vi "wait autonomous (WHS-ROB-6PZCBS1's conflicted copy 2013-02-20).vi"() -> ()   [LabVIEW 2010, in "Rampage.lvrbt"]
uses:
  Rampage.lvrbt
  <vilib>/NXT/Subs/MotorOutput.ctl
  <vilib>/NXT/NXTIO Xnodes/AddressXNode/NXTIOAddress.xnode
  <vilib>/NXT/Subs/MotorXNode.DC Motor Type.ctl
  <vilib>/NXT/Subs/MotorXNode.2DCMotor.ctl
  <vilib>/NXT/HiTechnic/HiTechnic Controls/HiTechnic Port.ctl
  <vilib>/NXT/Block Support/NXT_InputPort.ctl
  <vilib>/NXT/NXTIO Xnodes/NXTIOXNode/NXTIO.xnode
  <vilib>/NXT/Subs/LVHSConnector.ctl
  <vilib>/NXT/Dual Mode Library/Waits/Wait_Num(msec).vi
  <vilib>/NXT/Dual Mode Library/prims/inRangeAndCoerce/inRangeAndCoerce_int.vi
  <vilib>/NXT/Dual Mode Library/Motors/MotorOn.vi
  <vilib>/NXT/Dual Mode Library/Waits/Wait_Num.vi
  <vilib>/NXT/NXTIO Xnodes/NXTIONodeSubVIs/TETRIX IO Move DC Motors.vi
  <vilib>/NXT/NXTIO Xnodes/NXTIONodeSubVIs/TETRIX IO Stop DC Motors.vi
  <vilib>/NXT/Dual Mode Library/Sensors/Sonar_cm.vi
panel:
  out "Enabled":bool
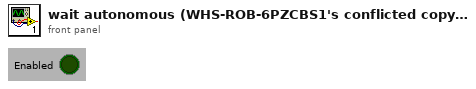
[diagram p1: front panel]
types:
  T1 = typedef "LVHSConnector.ctl" = cluster{"Hardware":string, "Flattened String":string}
  T2 = typedef "MotorOutput.ctl" = u8
  T3 = typedef "MotorXNode.DC Motor Type.ctl" = enum16{"DC Motor"}
  T4 = cluster{"DC Motor":T3, "Address":i16, "Address":i16}
  T5 = typedef "HiTechnic Port.ctl" = cluster{"Port":T6, "MUX Port":u8}
  T6 = typedef "NXT_InputPort.ctl" = u8
  T7 = cluster{"Direction (0-9)":i16, "Signal Strength (Array)":u8[]}
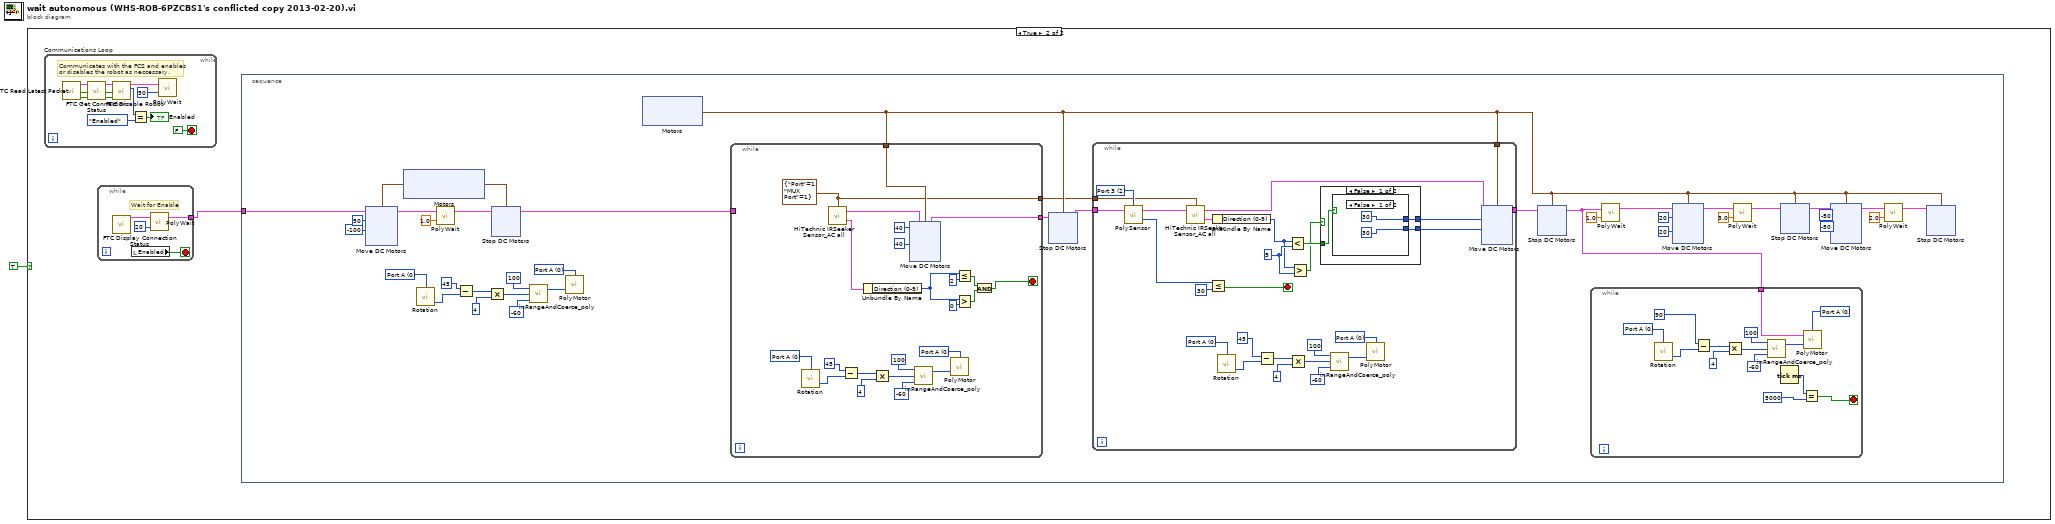
[diagram p0: block diagram]
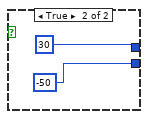
[diagram p3: hidden frame]
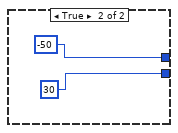
[diagram p4: hidden frame]
diagram:
  n1 = case shown="True" TRUE {
    frame False {
    }
    frame True {
      n2 = while "Communications Loop" {
        stop <- FALSE stop-if-true
        # "Communicates with the FCS and enables \nor disables the robot as neccessary."
        n3 = call <vilib>:"FTC Read Latest Packet.vi"() -> ("Packet Received?"=w213:bool, "Stopped?"=w212:bool, "NXT"=w215:T1)  [unwired: 6 in, 3 out]
        n4 = call <vilib>:"FTC Get Connection Status.vi"("Packet Received?"=w213, "Stopped?"=w212, "NXT"=w215) -> ("Online?"=w204:bool, "Stopped?"=w205:bool, "NXT"=w214:T1)  [unwired: 5 in]
        n5 = call <vilib>:"FTC Disable Robot.vi"("Online?"=w204, "Stopped?"=w205, "NXT"=w214) -> ("Enabled?"=w208:enum16{"Disabled", "Enabled"}, "NXT"=w210:T1)  [unwired: 3 in]
        n6 = Equal?(x=w208, y=enum16{"Disabled", "Enabled"}."Enabled") -> (x = y?=→"Enabled":bool)
        n7 = call-poly <vilib>:"PolyWait.vi"("Time (100 msec)"=u32 50 ("Time (msec)"), "NXT"=w210) -> ()  [unwired: 2 in, 1 out]
      }
      n8 = while {
        tunnel: [w201] -> w2
        stop <- w202 stop-if-true
        # "Wait for Enable"
        n9 = call <vilib>:"FTC Display Connection Status.vi"() -> ("NXT"=w200:T1)  [unwired: 11 in]
        n10 = local read "Enabled"() -> (w202:bool)
        n11 = call-poly <vilib>:"PolyWait.vi"("Time (100 msec)"=u32 20 ("Time (msec)"), "NXT"=w200) -> ("NXT"=w201:T1)  [unwired: 2 in]
      }
      n12 = stacked-sequence {
        tunnel: w2 -> [w4]
        frame #0 {
          w31 = T2 0 items=["Port A"=0, "Port B"=1, "Port C"=2, "Ports A & B"=4, "Ports A & C"=5, "Ports B & C"=6, "All Ports"=3] ("Output Port (All Ports)")
          w29 = u8 0 items=["Port A", "Port B", "Port C"] ("Port (Port A)")
          n13 = xnode "Motors"() -> ("DC Motor"=w39:T4)
          n14 = xnode "Move DC Motors"("Power/Speed 1"=i8 50, "Motors"=w39, "NXT"=w4, "Power/Speed 2"=i8 -100) -> ("NXT"=w37:T1)
          n15 = call <vilib>:"Rotation.vi"("Port (Port A)"=w29) -> ("Angle of Rotation"=w32:i32)  [unwired: 2 in, 1 out]
          n16 = call-poly <vilib>:"PolyWait.vi"("Time (1 sec)"=sgl 1.0, "NXT"=w37) -> ("NXT"=w34:T1)  [unwired: 2 in]
          n17 = Subtract(x=45 ("Claw\nPosition"), y=w32) -> (x-y=w30:i32)
          n18 = Multiply(x=w30, y=4) -> (x*y=w28:i32)
          n19 = xnode "Stop DC Motors"("Motors"=w39, "NXT"=w34) -> ("NXT"=w20:T1)
          n20 = call-poly <vilib>:"inRangeAndCoerce_poly.vi"("lower limit"=-60, "x"=w28, "upper limit"=100) -> ("coerced(x)"=w25:i32)  [unwired: 1 out]
          n21 = call-poly <vilib>:"PolyMotor.vi"("Power (75)"=w25, "Output Port (All Ports)"=w31) -> ()  [unwired: 2 in, 1 out]
          n22 = xnode "Motors"() -> ("DC Motor"=w22:T4)
          n23 = while {
            tunnel: [w188] -> w8
            tunnel: w22 -> [w185]
            tunnel: [w172] -> w3
            tunnel: w20 -> [_]
            stop <- w167 stop-if-true
            w177 = T2 0 items=["Port A"=0, "Port B"=1, "Port C"=2, "Ports A & B"=4, "Ports A & C"=5, "Ports B & C"=6, "All Ports"=3] ("Output Port (All Ports)")
            w179 = u8 0 items=["Port A", "Port B", "Port C"] ("Port (Port A)")
            w172 = T5 {"Port"=1, "MUX Port"=1} ("Port/MUX")
            n24 = call <vilib>:"Rotation.vi"("Port (Port A)"=w179) -> ("Angle of Rotation"=w176:i32)  [unwired: 2 in, 1 out]
            n25 = call <vilib>:"HiTechnic IRSeeker Sensor_AC all.vi"("Port/MUX"=w172) -> ("All Info"=w173:T7, "NXT"=w189:T1)  [unwired: 2 in]
            n26 = Subtract(x=45 ("Claw\nPosition"), y=w176) -> (x-y=w178:i32)
            n27 = Unbundle By Name(w173) -> ("Direction (0-9)"=w170:i16)
            n28 = Multiply(x=w178, y=4) -> (x*y=w180:i32)
            n29 = xnode "Move DC Motors"("Power/Speed 2"=i8 40, "Power/Speed 1"=i8 40, "Motors"=w185, "NXT"=w189) -> ("NXT"=w188:T1)
            n30 = call-poly <vilib>:"inRangeAndCoerce_poly.vi"("lower limit"=-60, "x"=w180, "upper limit"=100) -> ("coerced(x)"=w183:i32)  [unwired: 1 out]
            n31 = call-poly <vilib>:"PolyMotor.vi"("Power (75)"=w183, "Output Port (All Ports)"=w177) -> ()  [unwired: 2 in, 1 out]
            n32 = Less Or Equal?(x=w170, y=i16 2) -> (x <= y?=w169:bool)
            n33 = Greater?(x=w170, y=i16 0) -> (0:w168:bool)
            n34 = And(x=w169, y=w168) -> (x .and. y?=w167:bool)
          }
          n35 = xnode "Stop DC Motors"("Motors"=w22, "NXT"=w8) -> ("NXT"=w23:T1)
          n36 = while {
            tunnel: [w138] -> w7
            tunnel: w22 -> [w137]
            tunnel: w23 -> [w115]
            tunnel: w3 -> [w113]
            stop <- w114 stop-if-true
            w118 = T2 0 items=["Port A"=0, "Port B"=1, "Port C"=2, "Ports A & B"=4, "Ports A & C"=5, "Ports B & C"=6, "All Ports"=3] ("Output Port (All Ports)")
            w120 = u8 0 items=["Port A", "Port B", "Port C"] ("Port (Port A)")
            w129 = i16 5 ("y")
            w135 = T6 2 items=["Port 1", "Port 2", "Port 3", "Port 4"] ("Port (Port 4)")
            n37 = call-poly <vilib>:"PolySensor.vi"("NXT"=w115, "Port (Port 4)"=w135) -> ("Distance (cm)"=w136:i16, "NXT"=w134:T1)  [unwired: 1 in]
            n38 = call <vilib>:"HiTechnic IRSeeker Sensor_AC all.vi"("NXT"=w134, "Port/MUX"=w113) -> ("All Info"=w133:T7, "NXT"=w132:T1)  [unwired: 1 in]
            n39 = Less Or Equal?(x=w136, y=i16 30) -> (x <= y?=w114:bool)
            n40 = Unbundle By Name(w133) -> ("Direction (0-9)"=w128:i16)
            n41 = call <vilib>:"Rotation.vi"("Port (Port A)"=w120) -> ("Angle of Rotation"=w117:i32)  [unwired: 2 in, 1 out]
            n42 = Subtract(x=45 ("Claw\nPosition"), y=w117) -> (x-y=w119:i32)
            n43 = Less?(x=w128, y=w129) -> (x < y?=w127:bool)
            n44 = Multiply(x=w119, y=4) -> (x*y=w121:i32)
            n45 = Greater?(x=w128, y=w129) -> (0:w126:bool)
            n46 = case shown="False" w126 {
              tunnel: [w142 i8 -50 ("Power/Speed 2")] -> w131
              tunnel: [w141 i8 30 ("Power/Speed 1")] -> w130
              tunnel: w127 -> [w140 _]
              frame False {
                n47 = case shown="False" w140 {
                  tunnel: [i8 30 ("Power/Speed 1") i8 30 ("Power/Speed 2")] -> w142
                  tunnel: [i8 30 ("Power/Speed 2") i8 -50 ("Power/Speed 1")] -> w141
                  frame False {
                  }
                  frame True {
                  }
                }
              }
              frame True {
              }
            }
            n48 = call-poly <vilib>:"inRangeAndCoerce_poly.vi"("lower limit"=-60, "x"=w121, "upper limit"=100) -> ("coerced(x)"=w124:i32)  [unwired: 1 out]
            n49 = call-poly <vilib>:"PolyMotor.vi"("Power (75)"=w124, "Output Port (All Ports)"=w118) -> ()  [unwired: 2 in, 1 out]
            n50 = xnode "Move DC Motors"("Power/Speed 2"=w130, "Power/Speed 1"=w131, "Motors"=w137, "NXT"=w132) -> ("NXT"=w138:T1)
          }
          n51 = xnode "Stop DC Motors"("Motors"=w22, "NXT"=w7) -> ("NXT"=w21:T1)
          n52 = while {
            tunnel: w21 -> [w62]
            stop <- w59 stop-if-true
            w64 = T2 0 items=["Port A"=0, "Port B"=1, "Port C"=2, "Ports A & B"=4, "Ports A & C"=5, "Ports B & C"=6, "All Ports"=3] ("Output Port (All Ports)")
            w66 = u8 0 items=["Port A", "Port B", "Port C"] ("Port (Port A)")
            n53 = call <vilib>:"Rotation.vi"("Port (Port A)"=w66) -> ("Angle of Rotation"=w63:i32)  [unwired: 2 in, 1 out]
            n54 = Subtract(x=90 ("Claw\nPosition"), y=w63) -> (x-y=w65:i32)
            n55 = Multiply(x=w65, y=4) -> (x*y=w67:i32)
            n56 = call-poly <vilib>:"inRangeAndCoerce_poly.vi"("lower limit"=-60, "x"=w67, "upper limit"=100) -> ("coerced(x)"=w70:i32)  [unwired: 1 out]
            n57 = Tick Count (ms)() -> (millisecond timer value=w61:u32)
            n58 = Equal?(x=w61, y=u32 5000) -> (x = y?=w59:bool)
            n59 = call-poly <vilib>:"PolyMotor.vi"("Power (75)"=w70, "NXT"=w62, "Output Port (All Ports)"=w64) -> ()  [unwired: 1 in, 1 out]
          }
          n60 = call-poly <vilib>:"PolyWait.vi"("Time (1 sec)"=sgl 1.0, "NXT"=w21) -> ("NXT"=w19:T1)  [unwired: 2 in]
          n61 = xnode "Move DC Motors"("Power/Speed 2"=i8 20, "Power/Speed 1"=i8 20, "Motors"=w22, "NXT"=w19) -> ("NXT"=w11:T1)
          n62 = call-poly <vilib>:"PolyWait.vi"("Time (1 sec)"=sgl 3.0, "NXT"=w11) -> ("NXT"=w13:T1)  [unwired: 2 in]
          n63 = xnode "Stop DC Motors"("Motors"=w22, "NXT"=w13) -> ("NXT"=w14:T1)
          n64 = xnode "Move DC Motors"("Power/Speed 2"=i8 -50, "Power/Speed 1"=i8 -50, "Motors"=w22, "NXT"=w14) -> ("NXT"=w6:T1)
          n65 = call-poly <vilib>:"PolyWait.vi"("Time (1 sec)"=sgl 2.0, "NXT"=w6) -> ("NXT"=w15:T1)  [unwired: 2 in]
          n66 = xnode "Stop DC Motors"("Motors"=w22, "NXT"=w15) -> ()  [unwired: 1 out]
        }
      }
    }
  }
